vi "comunicacionvisaymega.vi"() -> ()   [LabVIEW 2015]
doc: "Uses the Match Pattern function to find all numbers in the given string, and returns them in an array. All of the following formats are recognized:\n\n123 1.23 .123 0.123 -1.23\n\nNo spaces or other characters may appear within the number, but any characters may appear before or after the number. This example assumes that the input string contains periods and not commas for the decimal separator."
panel:
  out "x*y":dbl
  out "element 2":dbl
  out "element":dbl
  out "Extracted Numbers":dbl[](array[numeric]) format="%#.6g"
  in  "String":string="one 2 -3 4.0 5.5"
  # "Overview: Demonstrates how to use the Match Pattern function to extract numeric values from a string.\nInstructions:\n1. Specify a String value containing numbers.\n2. Run the VI. All numbers in the String are displayed in the Extracted Numbers array."
  # "Note: Numbers that are spelled out (like \"one\" in the string above) are not interpreted as numbers.  Scientific notation is also not handled by this example. Additionally, this example will only extract decimal numbers from the string that use the \".\" character as a decimal separator."
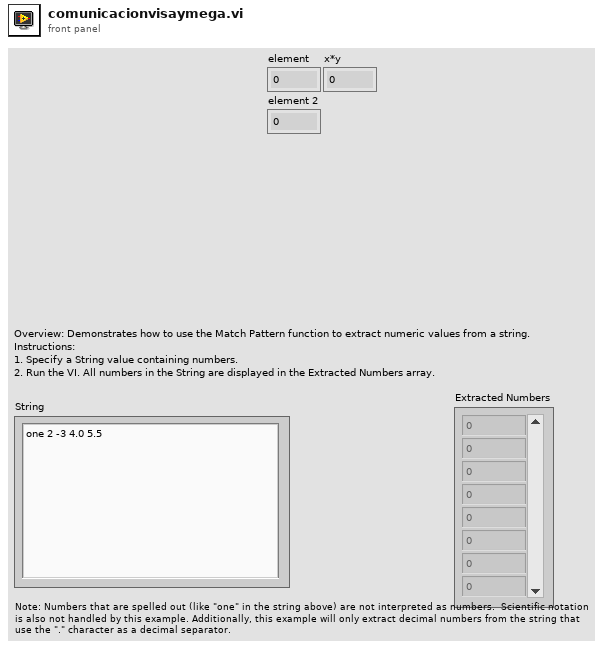
[diagram p1: front panel]
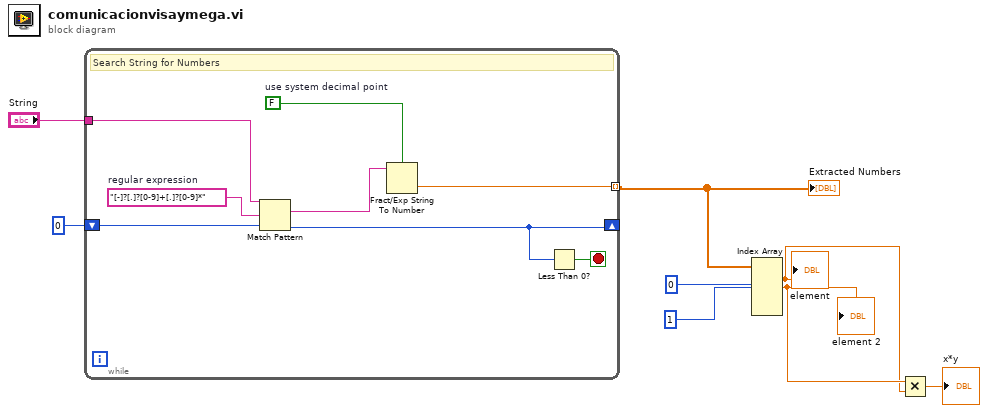
[diagram p0: block diagram]
diagram:
  n1 = while {
    tunnel: "String" -> [w16]
    shift-left: 0 -> [w13]
    shift-right: [w10] -> _
    tunnel: [w15] -> w4 mode=indexing
    stop <- w14 stop-if-true
    w12 = FALSE  # use system decimal point
    w9 = "[-]?[.]?[0-9]+[.]?[0-9]*"  # regular expression
    # "Search String for Numbers"
    n2 = Match Pattern(string=w16, regular expression=w9, offset (0)=w13) -> (match substring=w11:string, offset past match=w10:i32)  [unwired: 2 out]
    n3 = Fract/Exp String To Number(use system decimal point (T)=w12, string=w11) -> (number=w15:dbl)  [unwired: 2 in, 1 out]
    n4 = Less Than 0?(x=w10) -> (x < 0?=w14:bool)
  }
  "Extracted Numbers" <- w4
  n5 = Index Array(array=w4, index #1=0 ("index"), index #2=1 ("index")) -> (element #1=w2:dbl, element #2=w3:dbl)  [unwired: 3 in, 3 out]
  "element" <- w2
  "element 2" <- w3
  n6 = Multiply(x=w3, y=w2) -> (x*y=→"x*y":dbl)
